vi "Read Sync.vi"(8 "error in (no error)":errorcluster, 10 "Number Of Samples":i32, 11 "RTL-SDR in":refnum<class "RTL-SDR.lvclass">) -> (0 "error out":errorcluster, 1 "function return":i32, 2 "Sample Buffer":u8[](array[numeric]), 3 "RTL-SDR out":refnum<class "RTL-SDR.lvclass">, 4 "Samples Read":i32)   [LabVIEW 2015, in "RTL-SDR.lvclass"]
doc: "Created IvanLis by LabVIEW Portal\nProfile: http://labviewportal.org/memberlist.php?mode=viewprofile&u=987\neMail: IvanLisanov@gMail.com\nTelegram: https://t.me/IvanLis"
uses:
  RTL-SDR.lvclass
  RTL-SDR.lvclass/RTL-SDR.ctl
panel:
  in  "Samples Read In":i32
  in  "Sample Buffer In":u8[](array[numeric])
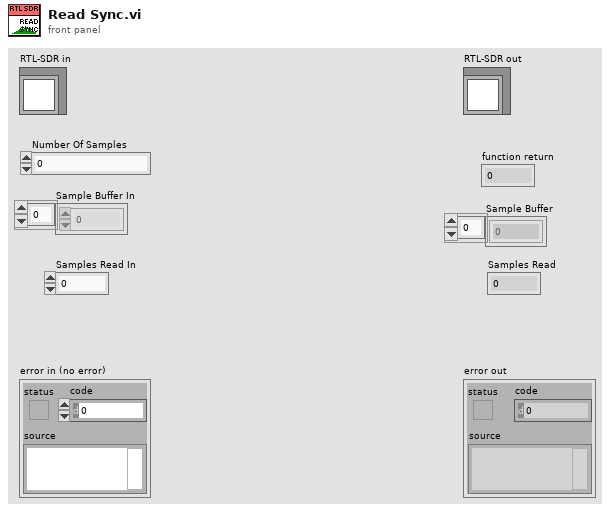
[diagram p1: front panel]
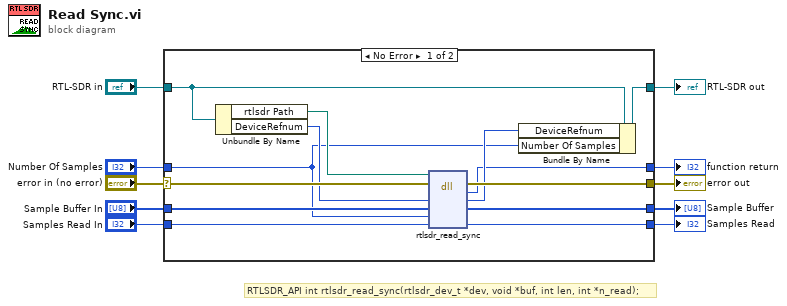
[diagram p0: block diagram]
diagram:
  # "RTLSDR_API int rtlsdr_read_sync(rtlsdr_dev_t *dev, void *buf, int len, int *n_read);"
  n1 = case shown="No Error" "error in (no error)" {
    selector: "error in (no error)" -> [w23 w25]
    tunnel: [w22 w25] -> w9
    tunnel: [w20 w24] -> w7
    tunnel: "RTL-SDR in" -> [w21 w24]
    tunnel: [w16 _] -> w6
    tunnel: "Sample Buffer In" -> [w15 _]
    tunnel: [w14 _] -> w4
    tunnel: "Number Of Samples" -> [w13 _]
    tunnel: "Samples Read In" -> [w12 _]
    tunnel: [w11 _] -> w1
    frame No Error {
      n2 = Unbundle By Name(w21) -> ("rtlsdr Path"=w19:path, "DeviceRefnum"=w18:u64)
      n3 = dll-call lib="C:/Users/Ivan/Desktop/D-23-09-24 (RTL-SDR)/Project (Pelleng-SDR)/rtlsdr/dll/rtlsdr.*" fn="rtlsdr_read_sync"(path in=w19, error in=w23, "DeviceRefnum"=w18, "SampleBuffer"=w15, "SamplesToRead"=w13, "SamplesRead"=w12) -> (error out=w22:errorcluster, "return type"=w16:i32, "DeviceRefnum"=w17:u64, "SampleBuffer"=w14:u8[], "SamplesRead"=w11:i32)  [unwired: 2 in, 1 out]
      n4 = Bundle By Name(cluster=w21, "DeviceRefnum"=w17, "Number Of Samples"=w13) -> (w20:refnum<class "RTL-SDR.lvclass">)
    }
    frame Error {
    }
  }
  "error out" <- w9
  "RTL-SDR out" <- w7
  "Samples Read" <- w1
  "Sample Buffer" <- w4
  "function return" <- w6
